vi "Write SP.vi"(8 "error in (no error)":errorcluster, 10 "SP":dbl, 11 "Generic Init CVT Message in":refnum<class "Generic Init CVT Message.lvclass">) -> (0 "error out":errorcluster, 3 "Generic Init CVT Message out":refnum<class "Generic Init CVT Message.lvclass">)   [LabVIEW 2014, in "DAQ Device.lvlib" / "Generic Init CVT Message.lvclass"]
uses:
  Generic Init CVT Message.lvclass
  Generic Init CVT Message.lvclass/Generic Init CVT Message.ctl
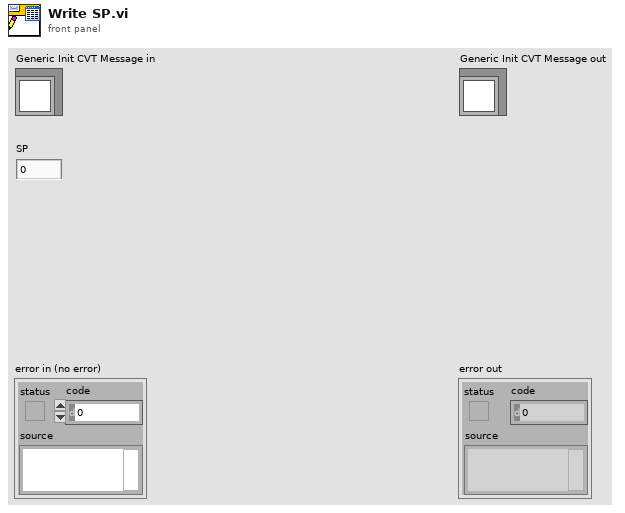
[diagram p1: front panel]
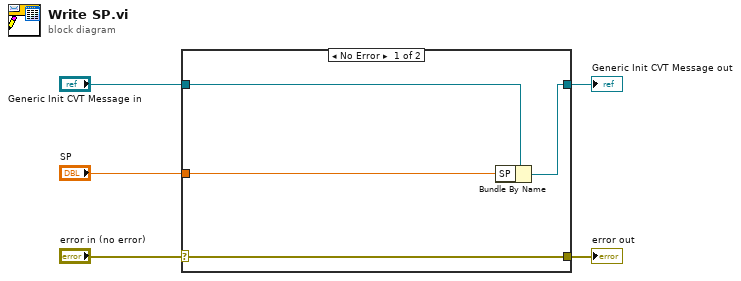
[diagram p0: block diagram]
diagram:
  n1 = case shown="No Error" "error in (no error)" {
    selector: "error in (no error)" -> [w9 w10]
    tunnel: [w9 w10] -> w4
    tunnel: [w7 w11] -> w2
    tunnel: "Generic Init CVT Message in" -> [w8 w11]
    tunnel: "SP" -> [w6 _]
    frame No Error {
      n2 = Bundle By Name(cluster=w8, "SP"=w6) -> (w7:refnum<class "Generic Init CVT Message.lvclass">)
    }
    frame Error {
    }
  }
  "error out" <- w4
  "Generic Init CVT Message out" <- w2
